vi "read_matrix_reshape_3D.vi"(10 "Dimensions":i32[](array[numeric]), 11 "Result in":dbl[][](array[numeric])) -> (3 "Result out":dbl[][][](array[numeric]))   [LabVIEW 2012]
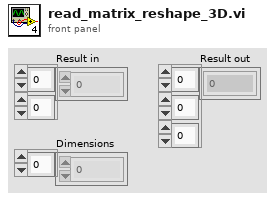
[diagram p1: front panel]
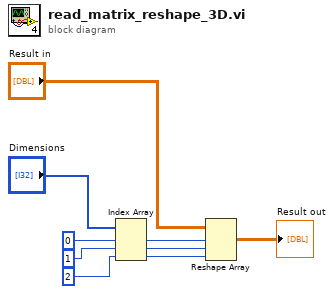
[diagram p0: block diagram]
diagram:
  n1 = Index Array(array="Dimensions", index #1=0 ("index"), index #2=1 ("index"), index #3=2 ("index")) -> (element #1=w6:i32, element #2=w7:i32, element #3=w8:i32)
  n2 = Reshape Array("Result in", w6, w7, w8) -> (→"Result out":dbl[][][])
